vi "Do.vi"(8 "error in (no error)":errorcluster, 10 "Actor in":refnum<class "Actor.lvclass">, 11 "Display Functions Message":refnum<class "Display Functions Message.lvclass">) -> (0 "error out":errorcluster, 2 "Actor out":refnum<class "Actor.lvclass">)   [LabVIEW 2016, in "Controller Actor.lvlib" / "Display Functions Message.lvclass"]
uses:
  <userlib>/Common Components/Controller/Messages/Populate Functions in UI/Display Functions Message.lvclass
  <vilib>/ActorFramework/Actor/Actor.lvclass
  <userlib>/Common Components/Controller/Controller.lvclass
  C:/Program Files (x86)/National Instruments/LabVIEW 2016/vi.lib/ActorFramework/Actor/Actor.lvclass
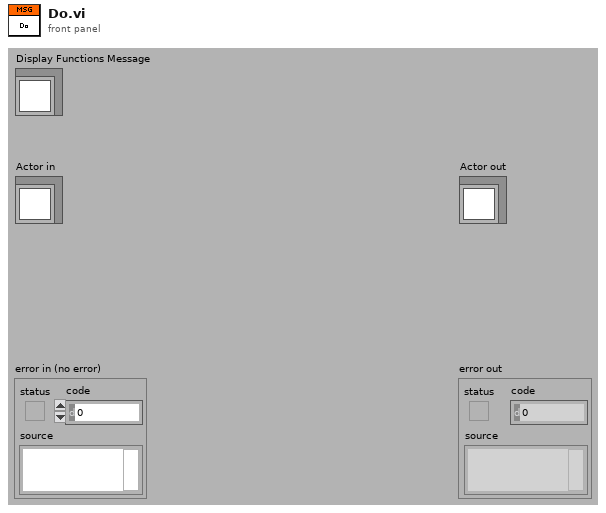
[diagram p1: front panel]
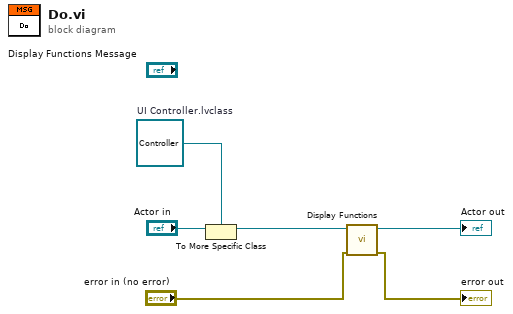
[diagram p0: block diagram]
diagram:
  w5 = refnum<class "Controller.lvclass"> refnum  # UI Controller.lvclass
  n1 = To More Specific Class(target class=w5, reference="Actor in") -> (specific class reference=w3:refnum<class "Controller.lvclass">)  [unwired: 1 in, 1 out]
  n2 = call <userlib>:"Display Functions.vi"("error in (no error)"="error in (no error)", "Controller in"=w3) -> ("error out"=→"error out":errorcluster, "Controller out"=→"Actor out":refnum<class "Controller.lvclass">)  [unwired: 8 in]
